vi "Single_Omit.vi"(3 "Accept In":bool[](array[boolean]), 4 "Data Values":string[](array[string]), 5 "Omit Strings":string[](array[string])) -> (0 "Accept Out":bool[](array[boolean]))   [LabVIEW 2018]
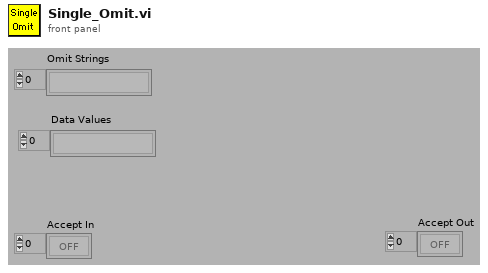
[diagram p1: front panel]
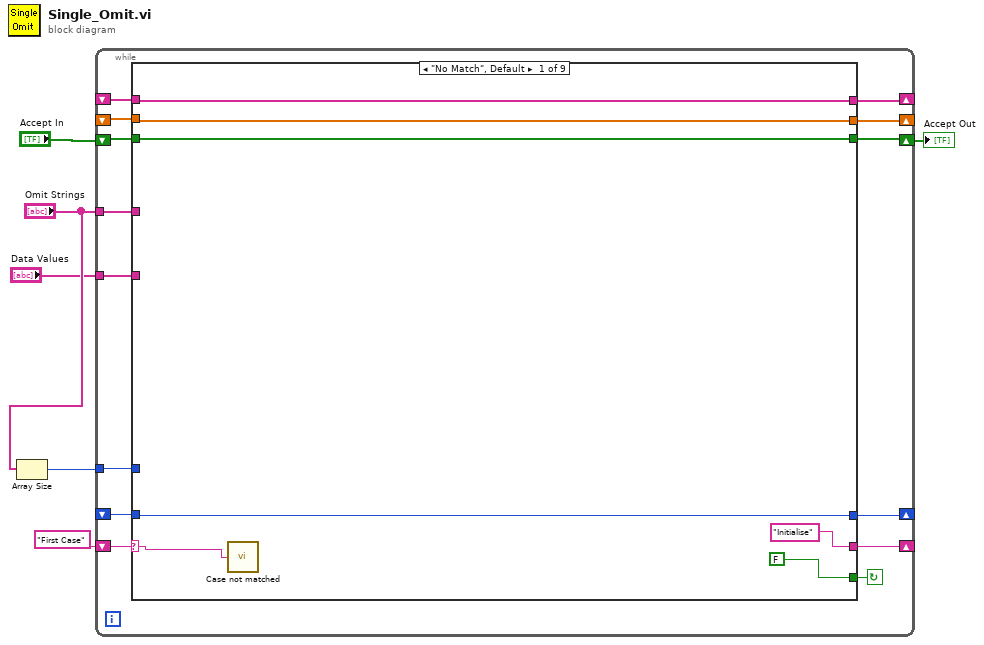
[diagram p0: block diagram]
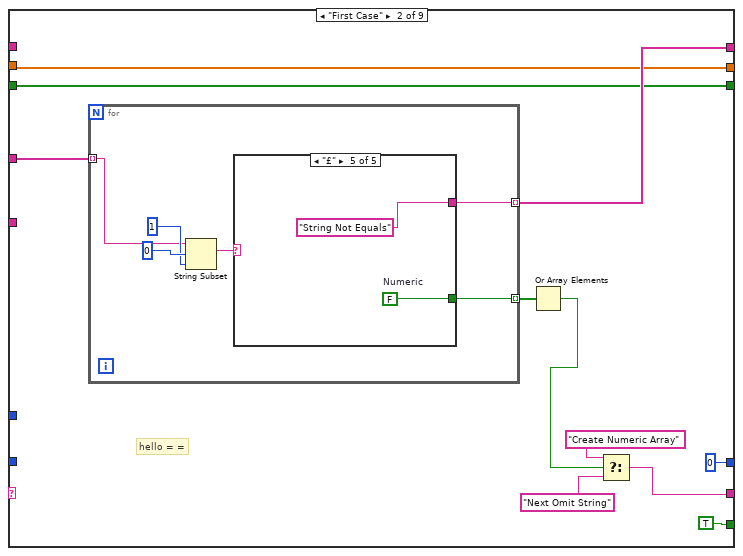
[diagram p2: hidden frame]
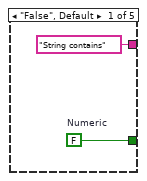
[diagram p3: hidden frame]
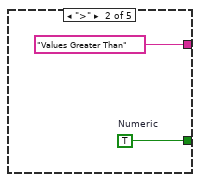
[diagram p4: hidden frame]
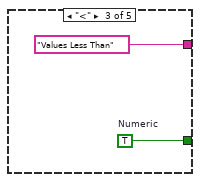
[diagram p5: hidden frame]
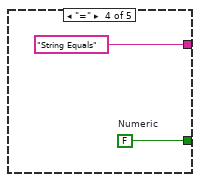
[diagram p6: hidden frame]
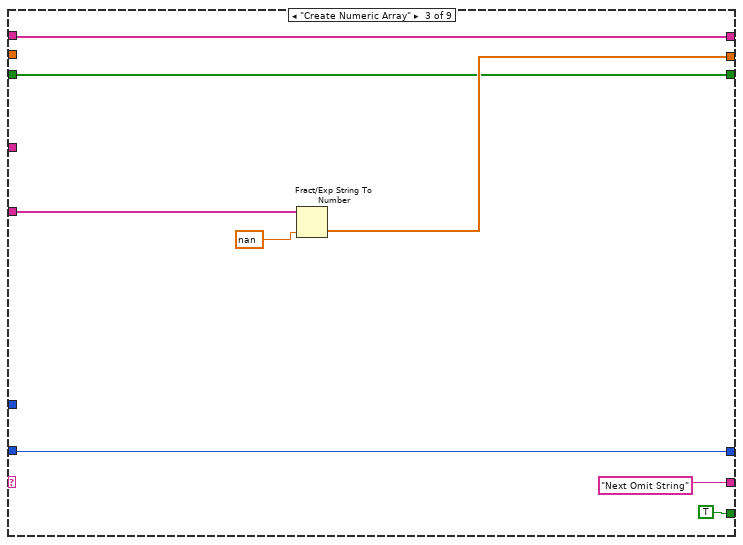
[diagram p7: hidden frame]
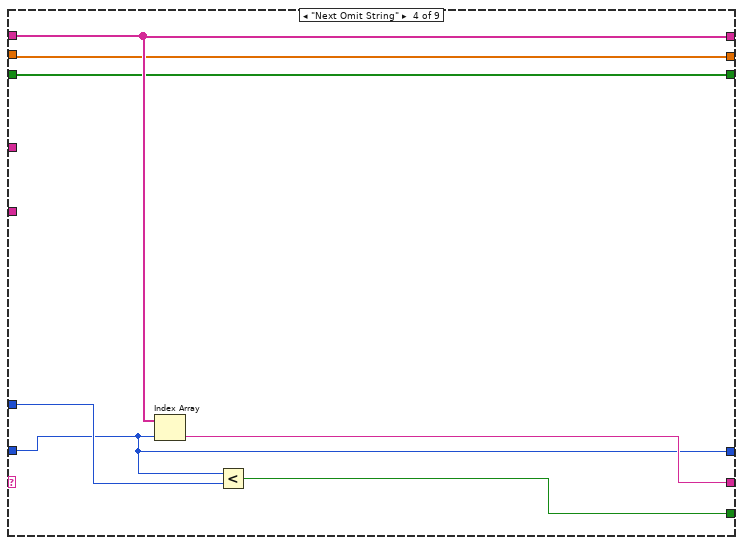
[diagram p8: hidden frame]
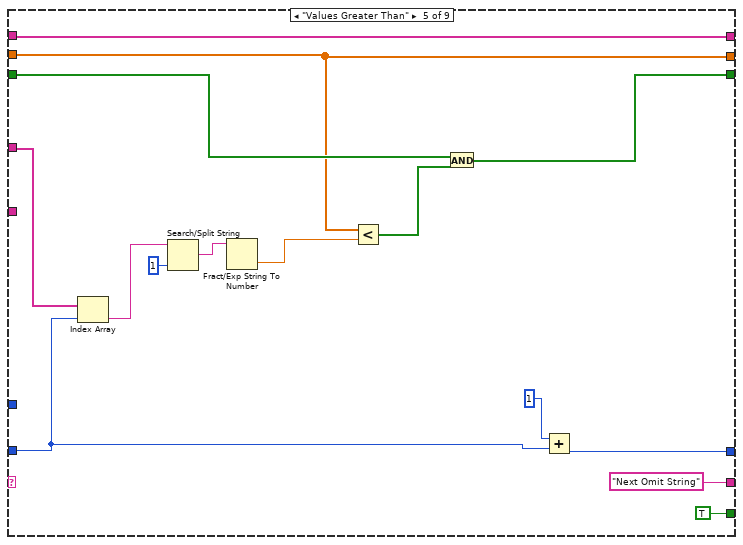
[diagram p9: hidden frame]
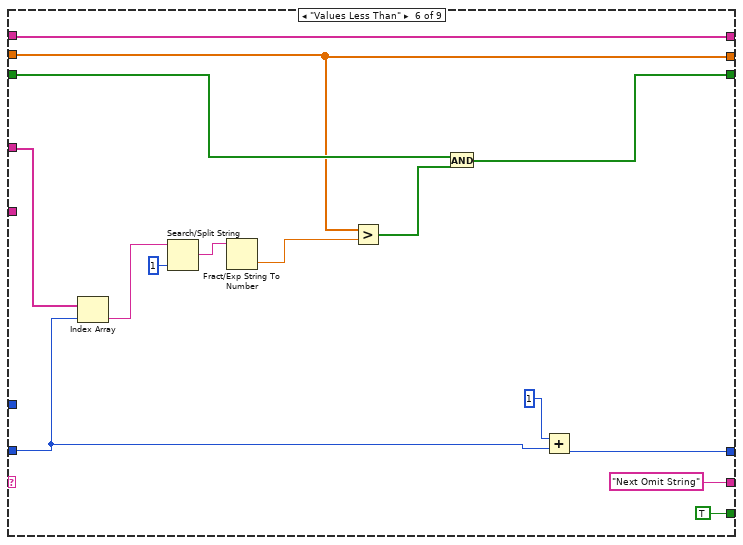
[diagram p10: hidden frame]
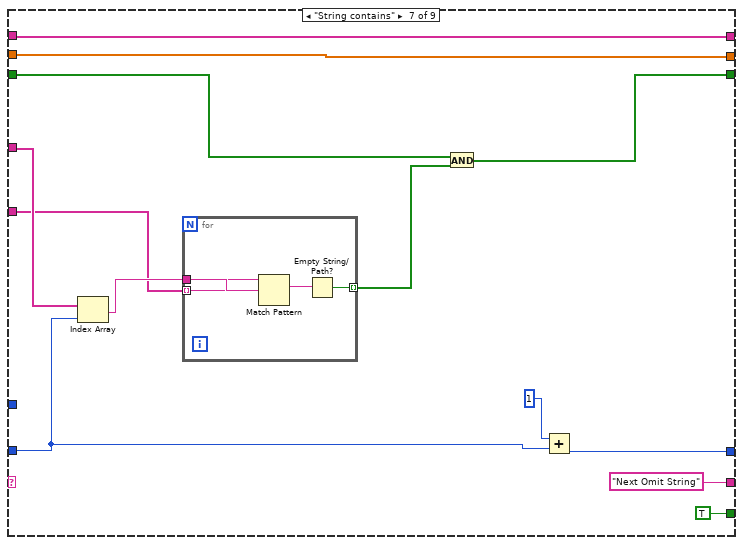
[diagram p11: hidden frame]
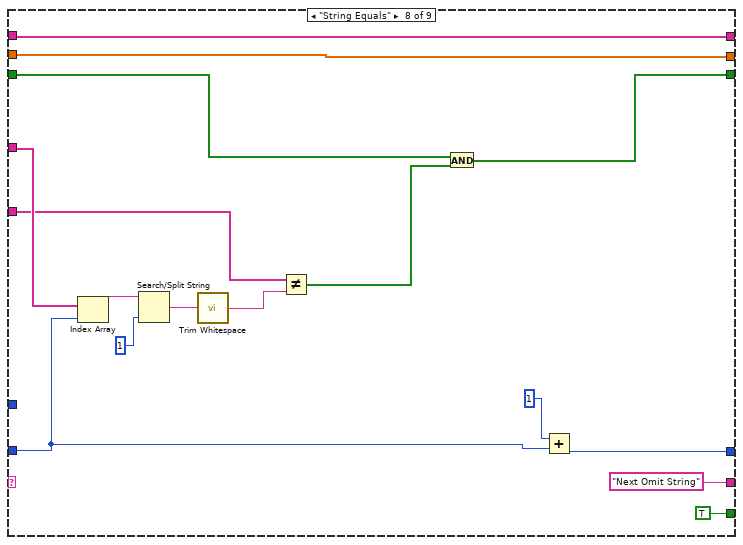
[diagram p12: hidden frame]
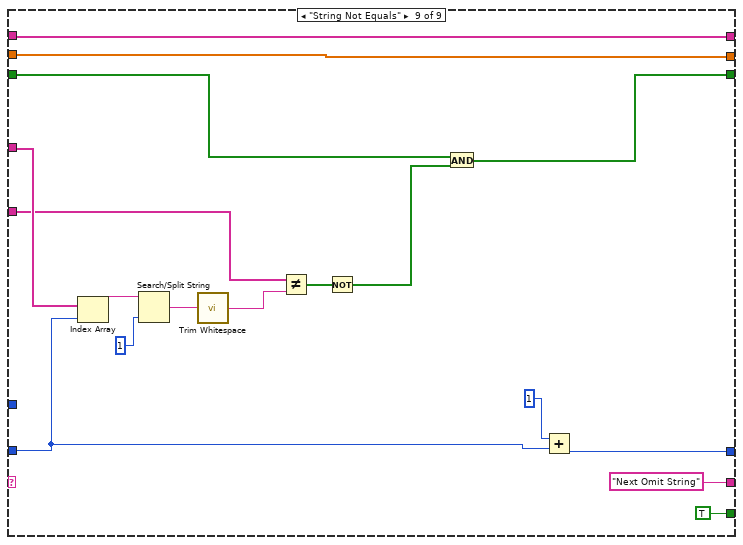
[diagram p13: hidden frame]
diagram:
  n1 = Array Size(array="Omit Strings") -> (size(s)=w3:i32)
  n2 = while {
    shift-left: "Accept In" -> [w7]
    shift-right: [w8] -> w2
    tunnel: w3 -> [w10]
    shift-left: _ -> [w9]
    shift-right: [w11] -> _
    tunnel: "Data Values" -> [w12]
    shift-left: _ -> [w13]
    shift-right: [w14] -> _
    tunnel: "Omit Strings" -> [w15]
    shift-left: _ -> [w17]
    shift-right: [w16] -> _
    shift-left: "First Case" -> [w18]
    shift-right: [w19] -> _
    stop <- w20 continue-if-true
    n3 = case shown="\"No Match\", Default" w18 {
      selector: w18 -> [w21 _ _ _ _ _ _ _ _]
      tunnel: [FALSE TRUE TRUE w68 TRUE TRUE TRUE TRUE TRUE] -> w20
      tunnel: ["Initialise" w31 "Next Omit String" w67 "Next Omit String" "Next Omit String" "Next Omit String" "Next Omit String" "Next Omit String"] -> w19
      tunnel: w17 -> [w25 _ w57 w65 w75 w90 w109 w129 w146]
      tunnel: [w25 w32 w57 w65 w75 w90 w109 w129 w146] -> w16
      tunnel: w15 -> [_ w37 _ _ w83 w98 w112 w132 w149]
      tunnel: [w22 0 w59 w66 w72 w87 w106 w126 w143] -> w14
      tunnel: w13 -> [w22 _ w59 w66 w74 w89 w108 w128 w145]
      tunnel: w12 -> [_ _ w61 _ _ _ w101 w118 w135]
      tunnel: [w24 w30 w60 w64 w76 w91 w103 w123 w140] -> w11
      tunnel: w10 -> [_ _ _ w69 _ _ _ _ _]
      tunnel: w9 -> [w24 w30 _ w64 w76 w91 w103 w123 w140]
      tunnel: [w23 w28 w56 w63 w77 w92 w110 w130 w147] -> w8
      tunnel: w7 -> [w23 w28 w56 w63 w78 w93 w111 w131 w148]
      frame "No Match", Default {
        n4 = call "Case not matched.vi"("Case Name not Matched"=w21) -> ()
      }
      frame "First Case" {
        # "hello = ="
        n5 = for {
          tunnel: w37 -> [w41] mode=indexing
          tunnel: [w40] -> w32 mode=indexing
          tunnel: [w39] -> w36 mode=indexing
          n6 = String Subset(string=w41, offset (0)=0, length (rest)=1 ("length")) -> (substring=w42:string)
          n7 = case shown="\"£\"" w42 {
            tunnel: ["String contains" "Values Greater Than" "Values Less Than" "String Equals" "String Not Equals"] -> w40
            tunnel: [w45 w47 w49 w51 w53] -> w39
            frame "False", Default {
              w45 = FALSE  # Numeric
            }
            frame ">" {
              w47 = TRUE  # Numeric
            }
            frame "<" {
              w49 = TRUE  # Numeric
            }
            frame "=" {
              w51 = FALSE  # Numeric
            }
            frame "£" {
              w53 = FALSE  # Numeric
            }
          }
        }
        n8 = Or Array Elements(Boolean array=w36) -> (logical OR=w35:bool)
        n9 = Select(t="Create Numeric Array", s=w35, f="Next Omit String") -> (s? t:f=w31:string)
      }
      frame "Create Numeric Array" {
        n10 = Fract/Exp String To Number(string=w61, default (0 dbl)=nan) -> (number=w60:dbl[])  [unwired: 3 out]
      }
      frame "Next Omit String" {
        n11 = Index Array(array=w65, index=w66) -> (element=w67:string)
        n12 = Less?(x=w66, y=w69) -> (x < y?=w68:bool)
      }
      frame "Values Greater Than" {
        n13 = Index Array(array=w83, index=w74) -> (element=w82:string)
        n14 = Search/Split String(string=w82, offset (0)=1) -> (match + rest of string=w81:string)  [unwired: 3 out]
        n15 = Fract/Exp String To Number(string=w81) -> (number=w80:dbl)  [unwired: 4 out]
        n16 = Less?(x=w76, y=w80) -> (x < y?=w79:bool[])
        n17 = And(x=w78, y=w79) -> (x .and. y?=w77:bool[])
        n18 = Add(x=1, y=w74) -> (x+y=w72:i32)
      }
      frame "Values Less Than" {
        n19 = Index Array(array=w98, index=w89) -> (element=w97:string)
        n20 = Search/Split String(string=w97, offset (0)=1) -> (match + rest of string=w96:string)  [unwired: 3 out]
        n21 = Fract/Exp String To Number(string=w96) -> (number=w95:dbl)  [unwired: 4 out]
        n22 = Greater?(x=w91, y=w95) -> (0:w94:bool[])
        n23 = And(x=w93, y=w94) -> (x .and. y?=w92:bool[])
        n24 = Add(x=1, y=w89) -> (x+y=w87:i32)
      }
      frame "String contains" {
        n25 = Index Array(array=w112, index=w108) -> (element=w102:string)
        n26 = for {
          tunnel: w102 -> [w116]
          tunnel: w101 -> [w115] mode=indexing
          tunnel: [w113] -> w100 mode=indexing
          n27 = Match Pattern(string=w115, regular expression=w116) -> (match substring=w114:string)  [unwired: 4 out]
          n28 = Empty String/Path?(string/path=w114) -> (empty?=w113:bool)
        }
        n29 = And(x=w111, y=w100) -> (x .and. y?=w110:bool[])
        n30 = Add(x=1, y=w108) -> (x+y=w106:i32)
      }
      frame "String Equals" {
        n31 = Index Array(array=w132, index=w128) -> (element=w121:string)
        n32 = Search/Split String(string=w121, offset (0)=1) -> (match + rest of string=w120:string)  [unwired: 3 out]
        n33 = call <vilib>:"Trim Whitespace.vi"("string"=w120) -> ("trimmed string"=w119:string)  [unwired: 1 in]
        n34 = Not Equal?(x=w118, y=w119) -> (x != y?=w117:bool[])
        n35 = And(x=w131, y=w117) -> (x .and. y?=w130:bool[])
        n36 = Add(x=1, y=w128) -> (x+y=w126:i32)
      }
      frame "String Not Equals" {
        n37 = Index Array(array=w149, index=w145) -> (element=w138:string)
        n38 = Search/Split String(string=w138, offset (0)=1) -> (match + rest of string=w137:string)  [unwired: 3 out]
        n39 = call <vilib>:"Trim Whitespace.vi"("string"=w137) -> ("trimmed string"=w136:string)  [unwired: 1 in]
        n40 = Not Equal?(x=w135, y=w136) -> (x != y?=w134:bool[])
        n41 = Not(x=w134) -> (.not. x?=w133:bool[])
        n42 = And(x=w148, y=w133) -> (x .and. y?=w147:bool[])
        n43 = Add(x=1, y=w145) -> (x+y=w143:i32)
      }
    }
  }
  "Accept Out" <- w2
